vi "Flatten.vi"(4 "T_Out":u64, 6 "T0":u64, 8 "error in (no error)":errorcluster, 10 "Data":T1[](array[typedef]), 11 "CIFTag in":refnum<class "CIF_NIChn_Fifo_Power.lvclass">) -> (0 "error out":errorcluster, 2 "Data out":T1[](array[typedef]), 3 "CIFTag out":refnum<class "CIF_NIChn_Fifo_Power.lvclass">)   [LabVIEW 2021, in "CIF_NIChn_Fifo_Power.lvclass"]
uses:
  CIF_NIChn_Fifo_Power.lvclass
  CIF_NIChn_Fifo_Power.lvclass/CIF_NIChn_Fifo_Power.ctl
  ChannelCommon/CIFFIFO/CIFfifo.lvclass
  ChannelCommon/typedef/Datatype Waveform.ctl
  ChannelCommon/ChannelCommon.lvlib
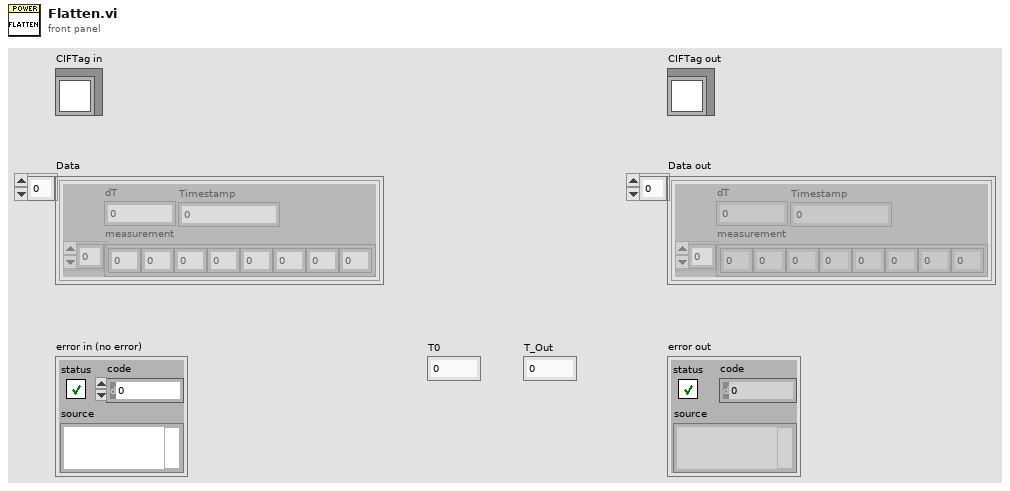
[diagram p1: front panel]
types:
  T1 = typedef "ChannelCommon.lvlib/Datatype Waveform.ctl" = cluster{"measurement":dbl[], "dT":dbl, "Timestamp":u64}
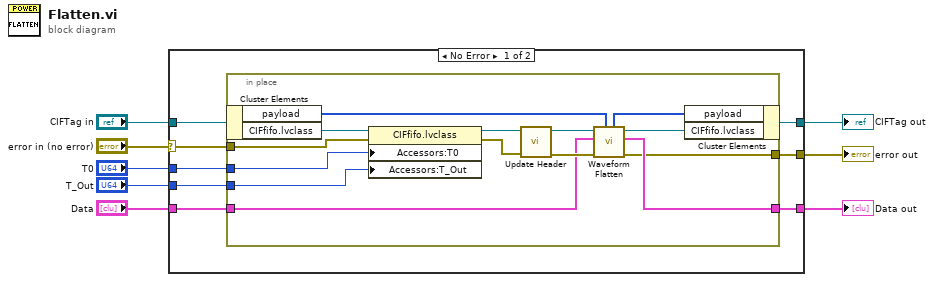
[diagram p0: block diagram]
diagram:
  n1 = case shown="No Error" "error in (no error)" {
    selector: "error in (no error)" -> [w9 w33]
    tunnel: [w14 w33] -> w7
    tunnel: [w13 w32] -> w5
    tunnel: "CIFTag in" -> [w10 w32]
    tunnel: "T_Out" -> [w16 _]
    tunnel: "T0" -> [w15 _]
    tunnel: "Data" -> [w12 w31]
    tunnel: [w11 w31] -> w1
    frame No Error {
      n2 = in-place {
        in-place-border: w16 -> [w27]
        in-place-border: w15 -> [w26]
        in-place-border: w9 -> [w25]
        in-place-border: [w17] -> w14
        in-place-border: w12 -> [w21]
        in-place-border: [w18] -> w11
        n3 = in-place-cluster #1(w10) -> ("payload"=w22:u8[], "CIFfifo.lvclass"=w30:refnum<class "CIFfifo.lvclass">)
        n4 = property class="CIFfifo.lvclass"(reference=w30, error in=w25, "Accessors:T0"=w26, "Accessors:T_Out"=w27) -> (reference out=w29:refnum<class "CIFfifo.lvclass">, error out=w28:errorcluster)
        n5 = call "Update Header.vi"("error in (no error)"=w28, "CIFFIFO in"=w29) -> ("error out"=w23:errorcluster, "CIFFIFO out"=w24:refnum<class "CIFfifo.lvclass">)  [unwired: 8 in]
        n6 = call "Waveform Flatten.vi"("payload in"=w22, "error in (no error)"=w23, "Data in"=w21, "CIFFifo in"=w24) -> ("error out"=w17:errorcluster, "Data out"=w18:T1[], "CIFFifo out"=w19:refnum<class "CIFfifo.lvclass">, "payload out"=w20:u8[])  [unwired: 3 in, 1 out]
        n7 = in-place-cluster #1("payload"=w20, "CIFfifo.lvclass"=w19) -> (w13:refnum<class "CIF_NIChn_Fifo_Power.lvclass">)
      }
    }
    frame Error {
    }
  }
  "error out" <- w7
  "CIFTag out" <- w5
  "Data out" <- w1
